vi "Initialize.vi"(8 "error in":errorcluster) -> (0 "error out":errorcluster)   [LabVIEW 2016, in "PLC.lvlib"]
uses:
  PLC.lvlib
  support/Message Queue/Message Queue.lvlib
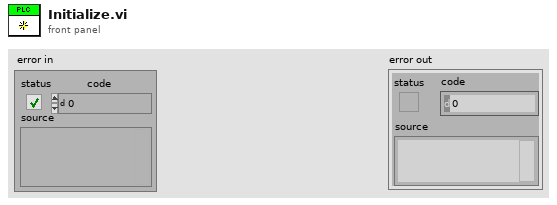
[diagram p1: front panel]
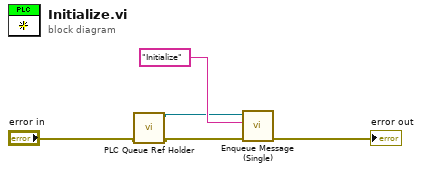
[diagram p0: block diagram]
diagram:
  n1 = call "PLC Queue Ref Holder.vi"("error in"="error in") -> ("error out"=w1:errorcluster, "Input Message Queue"=w2:refnum<queue>)  [unwired: 9 in]
  n2 = call "Enqueue Message (Single).vi"("error in (no error)"=w1, "Message"="Initialize", "Message Queue"=w2) -> ("error out"=→"error out":errorcluster)  [unwired: 7 in, 1 out]
